vi "tempo.vi"(11 "project-param out 3":T1) -> (3 "String":string)   [LabVIEW 2019]
uses:
  Project Parameters.ctl
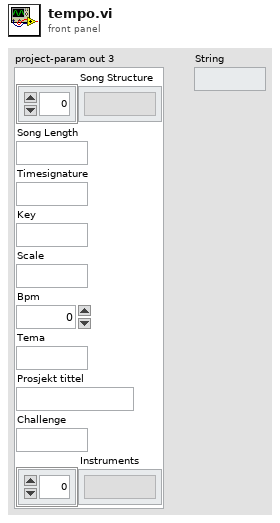
[diagram p1: front panel]
types:
  T1 = typedef "Project Parameters.ctl" = cluster{"Song Structure":string[], "Song Length":string, "Timesignature":string, "Key":string, "Scale":string, "Bpm":i32, "Tema":string, "Prosjekt tittel":string, "Challenge":string, "Instruments":string[]}
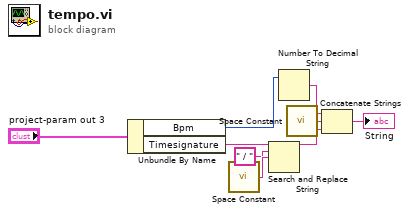
[diagram p0: block diagram]
diagram:
  n1 = Unbundle By Name("project-param out 3") -> ("Bpm"=w1:i32, "Timesignature"=w2:string)
  n2 = call <vilib>:"Space Constant.vi"() -> ("String"=w4:string)
  n3 = Search and Replace String(input string=w2, search string=" / ", replace string=w4) -> (result string=w8:string)  [unwired: 5 in, 3 out]
  n4 = Number To Decimal String(number=w1) -> (decimal integer string=w6:string)  [unwired: 1 in]
  n5 = call <vilib>:"Space Constant.vi"() -> ("String"=w7:string)
  n6 = Concatenate Strings(w6, w7, w8) -> (→"String":string)
